vi "DataCell_Tri.vi"(11 "Tableau 4":string[](array[string])) -> (1 "Tableau 2":dbl[][](array[numeric]), 2 "Tableau":string[](array[string]), 3 "Tableau 3":dbl[](array[numeric]))   [LabVIEW 2020]
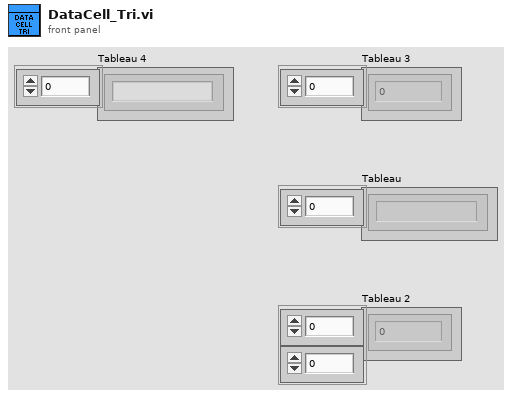
[diagram p1: front panel]
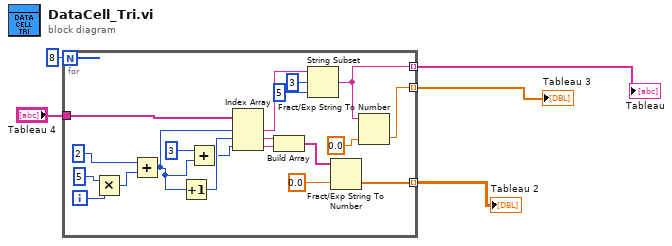
[diagram p0: block diagram]
diagram:
  n1 = for {
    N: 8 -> [_]
    tunnel: "Tableau 4" -> [w25]
    tunnel: [w13] -> w3 mode=indexing
    tunnel: [w12] -> w4 mode=indexing
    tunnel: [w6] -> w5 mode=indexing
    i -> [w23]
    n2 = Multiply(x=5, y=w23) -> (x*y=w22:i32)
    n3 = Add(x=2, y=w22) -> (x+y=w19:i32)
    n4 = Increment(x=w19) -> (x+1=w20:i32)
    n5 = Add(x=3, y=w19) -> (x+y=w17:i32)
    n6 = Index Array(array=w25, index #1=w19, index #2=w20, index #3=w17) -> (element #1=w9:string, element #2=w16:string, element #3=w15:string)
    n7 = Build Array(w16, w15) -> (w10:string[])
    n8 = String Subset(string=w9, offset (0)=3, length (rest)=5 ("longueur (reste)")) -> (substring=w6:string)
    n9 = Fract/Exp String To Number(string=w10, default (0 dbl)=0.0) -> (number=w12:dbl[])  [unwired: 2 in, 1 out]
    n10 = Fract/Exp String To Number(string=w6, default (0 dbl)=0.0) -> (number=w13:dbl)  [unwired: 2 in, 1 out]
  }
  "Tableau" <- w5
  "Tableau 2" <- w4
  "Tableau 3" <- w3
